vi "CreateWebServiceConfig.vi"   [LabVIEW 2015]
uses:
  <vilib>/AppBuilder/AB_Classes/RESTful/AB_RESTful_HTTPMethodType.ctl
  LabVIEW Server Source/Featherweight/Web/Server/FTW-WebService-IncomingRequestRouter.vi
  LabVIEW Server Source/Featherweight/Web/Server/FTW-WebService.lvclass
types:
  T1 = typedef "AB_RESTful_HTTPMethodType.ctl" = enum32{"GET", "POST", "PUT", "DELETE"}
  T2 = cluster{"Routing Template":string, "HTTP Verb":T1, "Callback VI Name":string}
  T3 = cluster{"Routing Template":string, "HTTP Verb":T1, "Callback VI Name":string}[]
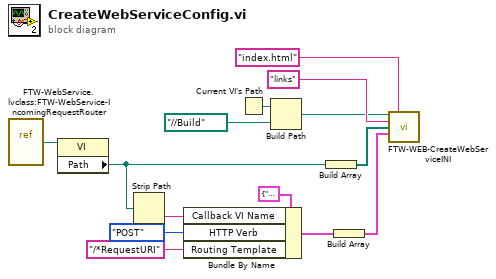
[diagram p0: block diagram]
diagram:
  n1 = vi-ref "FTW-WebService.lvclass:FTW-WebService-IncomingRequestRouter.vi"() -> (w5:refnum<vi>)
  n2 = property class="VI"(reference=w5) -> ("Path"=w4:path)  [unwired: 1 in, 2 out]
  n3 = Strip Path(path=w4) -> (name=w2:string)  [unwired: 1 out]
  n4 = Bundle By Name(cluster=T2 {"Routing Template"="", "HTTP Verb"=enum."GET", "Callback VI Name"=""} ("Routing Rule"), "Callback VI Name"=w2, "HTTP Verb"=AB_RESTful_HTTPMethodType."POST", "Routing Template"="/*RequestURI") -> (w9:T2)
  n5 = Current VI's Path() -> (path=w12:path)
  n6 = Build Path(base path=w12, name or relative path=path "../../Build") -> (appended path=w13:path)
  n7 = Build Array(w4) -> (w6:path[])
  n8 = Build Array(w9) -> (w8:T3)
  n9 = call "FTW-WEB-CreateWebServiceINI.vi"("Output Directory"=w13, "Default Document"="index.html", "Service Name"="links", "Request Handler Callback Filepaths"=w6, "Routing Rules"=w8) -> ()  [unwired: 9 in, 2 out]
